vi "DeQueue.vi"(8 "error in (no error)":errorcluster, 9 "Timeout":i32, 11 "queue ref":refnum<queue>) -> (0 "error out":errorcluster, 2 "State":string, 3 "queue out":refnum<queue>)   [LabVIEW 2022 SP3]
doc: "Use this template to build a VI to use as a subVI."
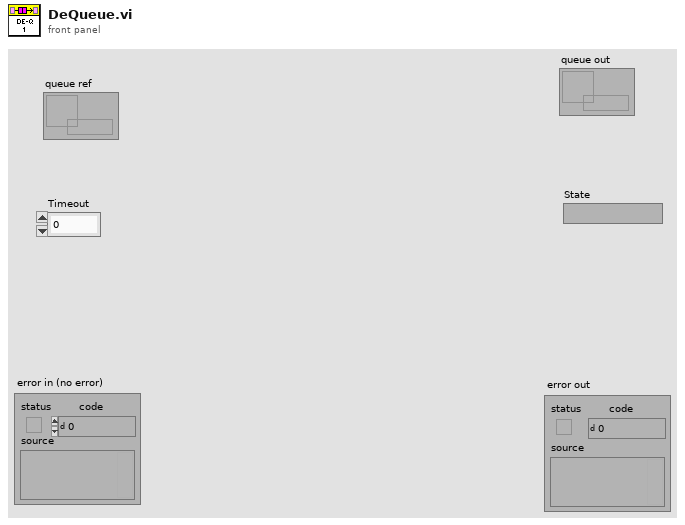
[diagram p1: front panel]
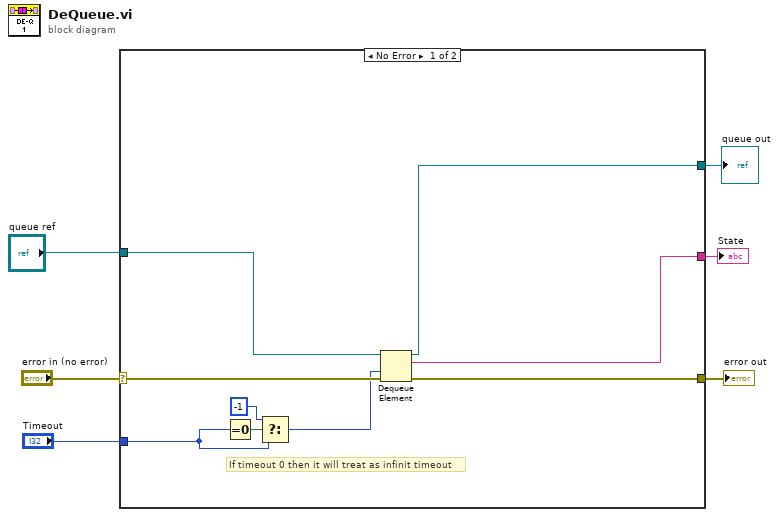
[diagram p0: block diagram]
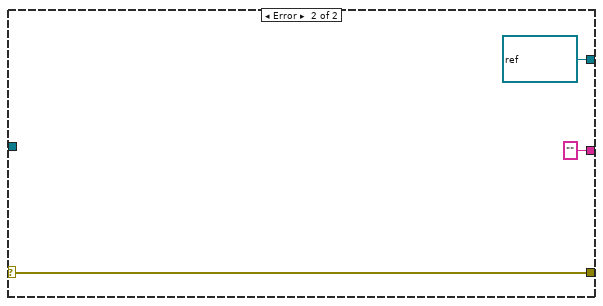
[diagram p2: hidden frame]
diagram:
  n1 = case shown="No Error" "error in (no error)" {
    selector: "error in (no error)" -> [w15 w18]
    tunnel: [w14 w18] -> w5
    tunnel: "queue ref" -> [w13 _]
    tunnel: "Timeout" -> [w10 _]
    tunnel: [w9 ""] -> w2
    tunnel: [w8 refnum<queue> refnum ("queue ref")] -> w1
    frame No Error {
      # "If timeout 0 then it will treat as infinit timeout"
      n2 = Equal To 0?(x=w10) -> (x = 0?=w12:bool)
      n3 = Select(t=-1, s=w12, f=w10) -> (s? t:f=w7:i32)
      n4 = Dequeue Element(queue=w13, timeout in ms (-1)=w7, error in (no error)=w15) -> (queue out=w8:refnum<queue>, element=w9:string, error out=w14:errorcluster)  [unwired: 1 out]
    }
    frame Error {
    }
  }
  "error out" <- w5
  "State" <- w2
  "queue out" <- w1
